vi "Day 9-Pad Array.vi"(11 "Array in":i32[][](array[numeric])) -> (3 "Array out":i32[][](array[numeric]))   [LabVIEW 2021]
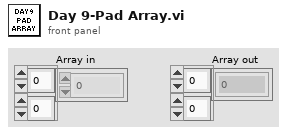
[diagram p1: front panel]
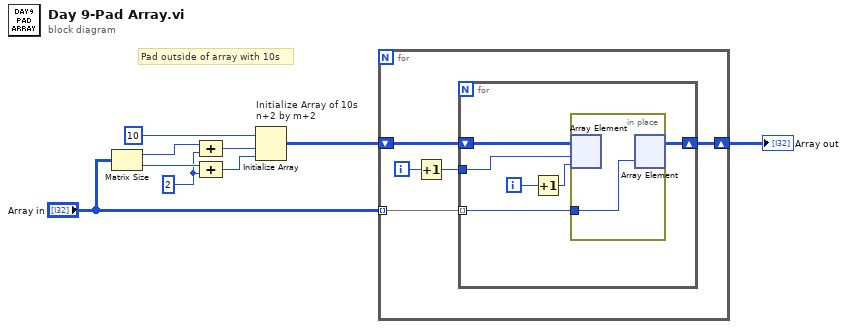
[diagram p0: block diagram]
diagram:
  w4 = 2 ("value")
  # "Pad outside of array with 10s"
  n1 = Matrix Size(0:"Array in") -> (1:w8:i32, 2:w6:i32)
  n2 = Compound Arithmetic op=ADD(w8, w4) -> (w9:i32)
  n3 = Compound Arithmetic op=ADD(w6, w4) -> (w7:i32)
  n4 = Initialize Array "Initialize Array of 10s\nn+2 by m+2"(10, w9, w7) -> (w5:i32[][])
  n5 = for {
    tunnel: "Array in" -> [w11] mode=indexing
    shift-right: [w10] -> w1
    shift-left: w5 -> [w14]
    i -> [w13]
    n6 = Increment(x=w13) -> (x+1=w12:i32)
    n7 = for {
      tunnel: w12 -> [w19]
      tunnel: w11 -> [w17] mode=indexing
      shift-right: [w15] -> w10
      shift-left: w14 -> [w20]
      i -> [w18]
      n8 = Increment(x=w18) -> (x+1=w16:i32)
      n9 = in-place {
        in-place-border: w17 -> [w21]
        n10 = in-place-array #1(w20, w19, w16) -> ()  [unwired: 1 out]
        n11 = in-place-array #1(w21) -> (w15:i32[][])  [unwired: 2 out]
      }
    }
  }
  "Array out" <- w1
